vi "Write.vi"(8 "error in (no error)":errorcluster, 10 "write buffer":string, 11 "VGC in":refnum<class "PL Inficon VGC.lvclass">) -> (0 "error out":errorcluster, 3 "VGC out":refnum<class "PL Inficon VGC.lvclass">)   [LabVIEW 2015, in "PL Inficon VGC.lvclass"]
doc: "Writes bytes to specified interface."
uses:
  PL Inficon VGC.lvclass
  PL Inficon VGC.lvclass/PL Inficon VGC.ctl
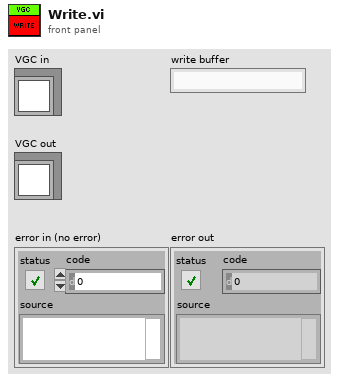
[diagram p1: front panel]
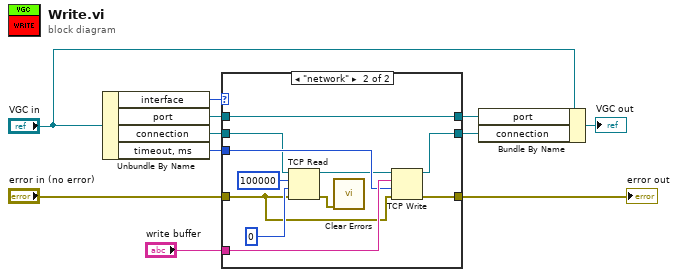
[diagram p0: block diagram]
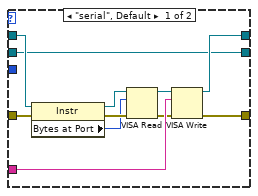
[diagram p2: hidden frame]
diagram:
  n1 = Unbundle By Name("VGC in") -> ("interface"=w10:enum16{"serial", "network"}, "port"=w9:refnum<visa-resource-name>, "connection"=w8:refnum<k5>, "timeout, ms"=w6:u32)
  n2 = case shown="\"network\"" w10 {
    tunnel: "error in (no error)" -> [w16 w26]
    tunnel: [w22 w33] -> w1
    tunnel: "write buffer" -> [w21 w32]
    tunnel: w9 -> [w14 w31]
    tunnel: w8 -> [w12 w25]
    tunnel: [w13 w31] -> w4
    tunnel: w6 -> [_ w30]
    tunnel: [w12 w29] -> w3
    frame "serial", Default {
      n3 = property class="Instr"(reference=w14, error in=w16) -> (reference out=w19:refnum<visa-resource-name>, error out=w18:errorcluster, "Bytes at Port"=w17:u32)
      n4 = VISA Read(VISA resource name=w19, byte count=w17, error in (no error)=w18) -> (VISA resource name out=w20:refnum<visa-resource-name>, error out=w15:errorcluster)  [unwired: 2 out]
      n5 = VISA Write(VISA resource name=w20, write buffer=w21, error in (no error)=w15) -> (VISA resource name out=w13:refnum<visa-resource-name>, error out=w22:errorcluster)  [unwired: 1 out]
    }
    frame "network" {
      n6 = TCP Read(connection ID=w25, bytes to read=100000, error in (no error)=w26, 9:0 ("timeout ms (25000)")) -> (connection ID out=w24:refnum<k5>, error out=w23:errorcluster)  [unwired: 1 in, 1 out]
      n7 = call <vilib>:"Clear Errors.vi"("error in (no error)"=w23) -> ()  [unwired: 5 in, 2 out]
      n8 = TCP Write(connection ID=w24, data in=w32, error in (no error)=w26, 9:w30) -> (connection ID out=w29:refnum<k5>, error out=w33:errorcluster)  [unwired: 1 out]
    }
  }
  "error out" <- w1
  n9 = Bundle By Name(cluster="VGC in", "port"=w4, "connection"=w3) -> (→"VGC out":refnum<class "PL Inficon VGC.lvclass">)
